vi "Value String to Value Variant.vi"(9 "Type Descriptor Enumeration":T1 format="%.0x", 10 "Default":variant, 11 "Value String":string) -> (3 "Value Variant":variant)   [LabVIEW 2016]
uses:
  <userlib>/_OpenG.lib/lvdata/lvdata.llb/Type Descriptor Enumeration__ogtk.ctl
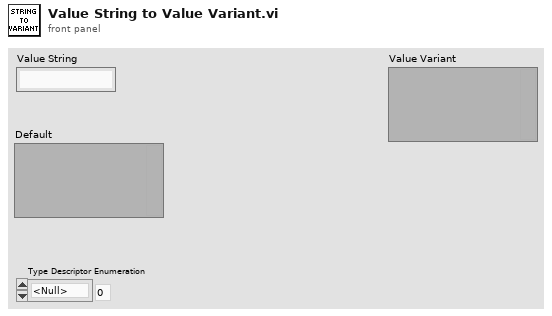
[diagram p1: front panel]
types:
  T1 = typedef "Type Descriptor Enumeration__ogtk.ctl" = enum8{"<Null>", "I8", "I16", "I32", "I64", "U8", "U16", "U32", "U64", "SGL", "DBL", "EXT", "CSG", "CDB", "CXT", "0x0F", "0x10", "0x11", "0x12", "0x13", "0x14", "Enum U8", "Enum U16", "Enum U32", "Enum U64", "SGL PQ", "DBL PQ", "EXT PQ", "CSG PQ", "CDB PQ", "CXT PQ", "0x1F", "0x20", "Boolean", "0x22", "0x23", "0x24", "0x25", "0x26", "0x27", "0x28", "0x29", "0x2A", "0x2B", "0x2C", "0x2D", "0x2E", "0x2F", "String", "0x31", "Path", "Pict", "0x34", "0x35", "0x36", "DAQ", "0x38", "0x39", "0x3A", "0x3B", "0x3C", "0x3D", "0x3E", "0x3F", "Array", "0x41", "0x42", "0x43", "0x44", "0x45", "0x46", "0x47", "0x48", "0x49", "0x4A", "0x4B", "0x4C", "0x4D", "0x4E", "0x4F", "Cluster", "0x51", "0x52", "Variant", "Waveform", "0x55", "0x56", "0x57", "0x58", "0x59", "0x5A", "0x5B", "0x5C", "0x5D", "0x5E", "0x5F", "0x60", "0x61", "0x62", "0x63", "0x64", "0x65", "0x66", "0x67", "0x68", "0x69", "0x6A", "0x6B", "0x6C", "0x6D", "0x6E", "0x6F", "Refnum"}
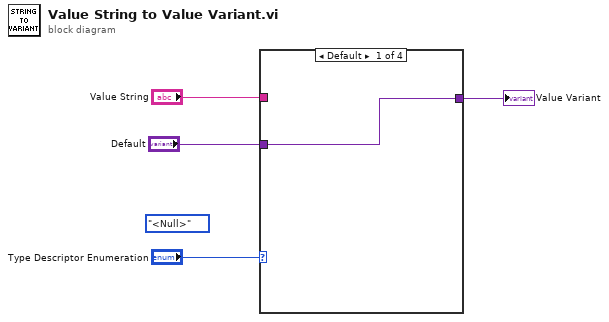
[diagram p0: block diagram]
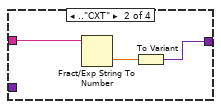
[diagram p2: hidden frame]
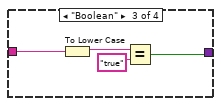
[diagram p3: hidden frame]
diagram:
  (unwired) Type_Descriptor_Enumeration__ogtk."<Null>" ("Type Descriptor Enumeration")
  n1 = case shown="Default" "Type Descriptor Enumeration" {
    tunnel: "Value String" -> [_ w8 w12 w13]
    tunnel: [w5 w6 w9 w13] -> w3
    tunnel: "Default" -> [w5 _ _ _]
    frame Default {
    }
    frame .."CXT" {
      n2 = Fract/Exp String To Number(string=w8) -> (number=w7:dbl)  [unwired: 3 in, 1 out]
      n3 = To Variant(anything=w7) -> (Variant=w6:variant)
    }
    frame "Boolean" {
      n4 = To Lower Case(string=w12) -> (all lower case string=w11:string)
      n5 = Equal?(x=w11, y="true") -> (x = y?=w9:bool)
    }
    frame "String" {
    }
  }
  "Value Variant" <- w3
